vi "Timestamp T_Out Control.vi"(6 "Disable FIFO Out Benchmark":bool, 8 "error in (no error)":errorcluster, 10 "Logic Sleep Stats":T1={"Target Wake Time"=0, "Wake Time"=0, "Sleep TIme"=0, "Timeout (Housekeep)"=TRUE, "T_Out (ns)"=0}, 11 "CIFCorePlugin in":refnum<class "CIFCorePlugin.lvclass">) -> (0 "error out":errorcluster, 3 "CIFCorePlugin out":refnum<class "CIFCorePlugin.lvclass">)   [LabVIEW 2021, in "CIFCorePlugin.lvclass"]
doc: "This can be used to provide timestamps for plugin benchmarks if skip sleep is true and timing (and sleep) is controlled directly in the logic block. It will update timestamps each time it is called."
uses:
  CIFCorePlugin.lvclass
  Typedef/Logic Sleep Stats.ctl
  CIFCorePlugin.lvclass/CIFCorePlugin.ctl
  <vilib>/CIF Foundation/CIF Utilities/Time/System Time/Get System Time.vi
  <vilib>/CIF Foundation/CIF Utilities/Time/System Time/LabVIEW Time to TAI Time.vi
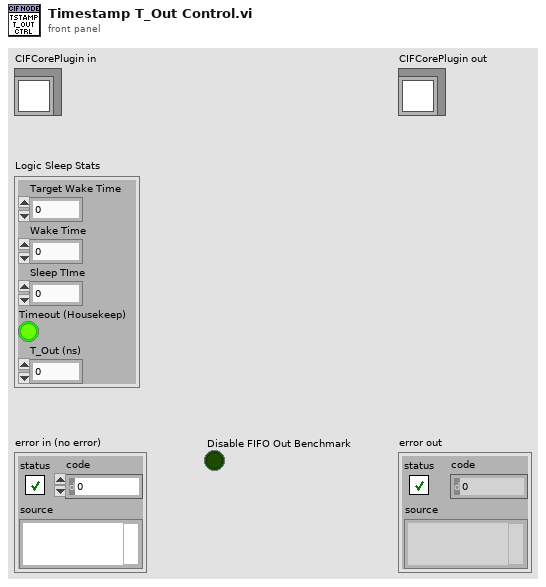
[diagram p1: front panel]
types:
  T1 = typedef "CIFCorePlugin.lvclass/Logic Sleep Stats.ctl" = cluster{"Target Wake Time":i64, "Wake Time":i64, "Sleep TIme":i64, "Timeout (Housekeep)":bool, "T_Out (ns)":i64}
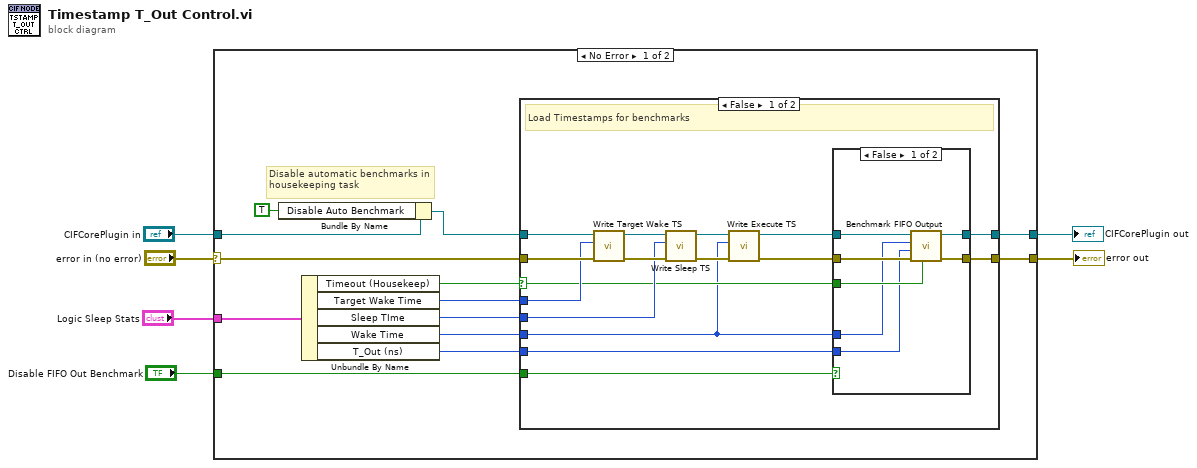
[diagram p0: block diagram]
diagram:
  n1 = case shown="No Error" "error in (no error)" {
    selector: "error in (no error)" -> [w19 w48]
    tunnel: [w17 w48] -> w3
    tunnel: [w18 w47] -> w4
    tunnel: "CIFCorePlugin in" -> [w16 w47]
    tunnel: "Logic Sleep Stats" -> [w13 _]
    tunnel: "Disable FIFO Out Benchmark" -> [w7 _]
    frame No Error {
      # "Disable automatic benchmarks in housekeeping task"
      n2 = Bundle By Name(cluster=w16, "Disable Auto Benchmark"=TRUE ("Running Internal Data.Disable Auto Benchmark")) -> (w14:refnum<class "CIFCorePlugin.lvclass">)
      n3 = Unbundle By Name(w13) -> ("Timeout (Housekeep)"=w12:bool, "Target Wake Time"=w9:i64, "Sleep TIme"=w10:i64, "Wake Time"=w11:i64, "T_Out (ns)"=w8:i64)
      n4 = case shown="False" w12 {
        selector: w12 -> [w23 _]
        tunnel: w19 -> [w34 w45]
        tunnel: [w25 w46] -> w18
        tunnel: [w24 w45] -> w17
        tunnel: w14 -> [w35 w46]
        tunnel: w11 -> [w21 _]
        tunnel: w10 -> [w29 _]
        tunnel: w9 -> [w28 _]
        tunnel: w8 -> [w22 _]
        tunnel: w7 -> [w20 _]
        frame False {
          # "Load Timestamps for benchmarks"
          n5 = call "Write Target Wake TS.vi"("error in (no error)"=w34, "Target Wake"=w28, "CIFCorePlugin in"=w35) -> ("error out"=w30:errorcluster, "CIFCorePlugin out"=w33:refnum<class "CIFCorePlugin.lvclass">)  [unwired: 7 in]
          n6 = call "Write Sleep TS.vi"("error in (no error)"=w30, "Sleep"=w29, "CIFCorePlugin in"=w33) -> ("error out"=w31:errorcluster, "CIFCorePlugin out"=w32:refnum<class "CIFCorePlugin.lvclass">)  [unwired: 7 in]
          n7 = call "Write Execute TS.vi"("error in (no error)"=w31, "Execute"=w21, "CIFCorePlugin in"=w32) -> ("error out"=w26:errorcluster, "CIFCorePlugin out"=w27:refnum<class "CIFCorePlugin.lvclass">)  [unwired: 7 in]
          n8 = case shown="False" w20 {
            tunnel: w27 -> [w42 w44]
            tunnel: w26 -> [w41 w43]
            tunnel: [w40 w44] -> w25
            tunnel: [w39 w43] -> w24
            tunnel: w23 -> [w38 _]
            tunnel: w22 -> [w37 _]
            tunnel: w21 -> [w36 _]
            frame False {
              n9 = call "Benchmark FIFO Output.vi"("timed out?"=w38, "error in (no error)"=w41, "T_Out"=w37, "T_Write"=w36, "CIFCorePlugin in"=w42) -> ("error out"=w39:errorcluster, "CIFCorePlugin out"=w40:refnum<class "CIFCorePlugin.lvclass">)  [unwired: 5 in]
            }
            frame True {
            }
          }
        }
        frame True {
          # "Housekeep only"
        }
      }
    }
    frame Error {
    }
  }
  "error out" <- w3
  "CIFCorePlugin out" <- w4
